vi "_GUI Template.vi"(8 "error in":errorcluster) -> (0 "error out":errorcluster)   [LabVIEW 2010]
doc: "GUI"
uses:
  <vilib>/Utility/miscctls.llb/LVPointTypeDef.ctl
panel:
  in  "Cancel":bool
  in  "OK":bool
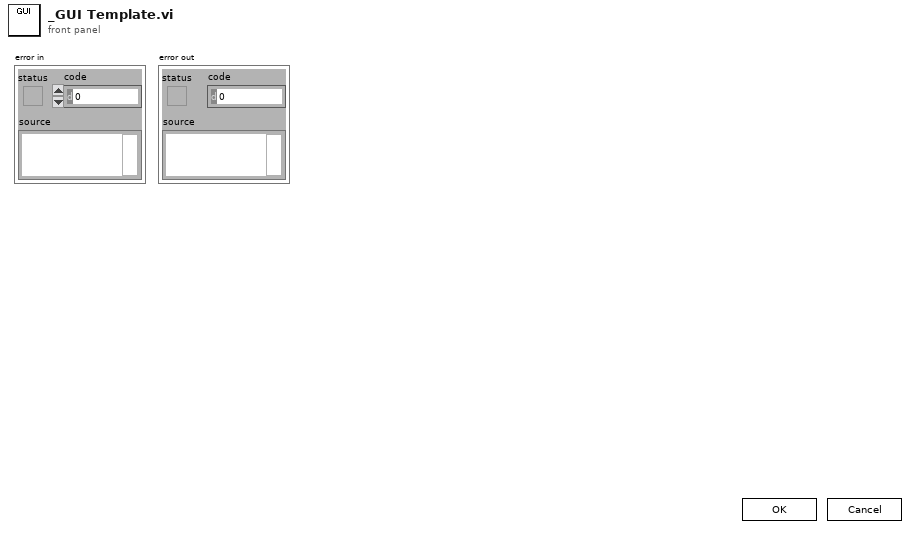
[diagram p1: front panel]
types:
  T1 = typedef "LVPointTypeDef.ctl" = cluster{"Horizontal":i16, "Vertical":i16}
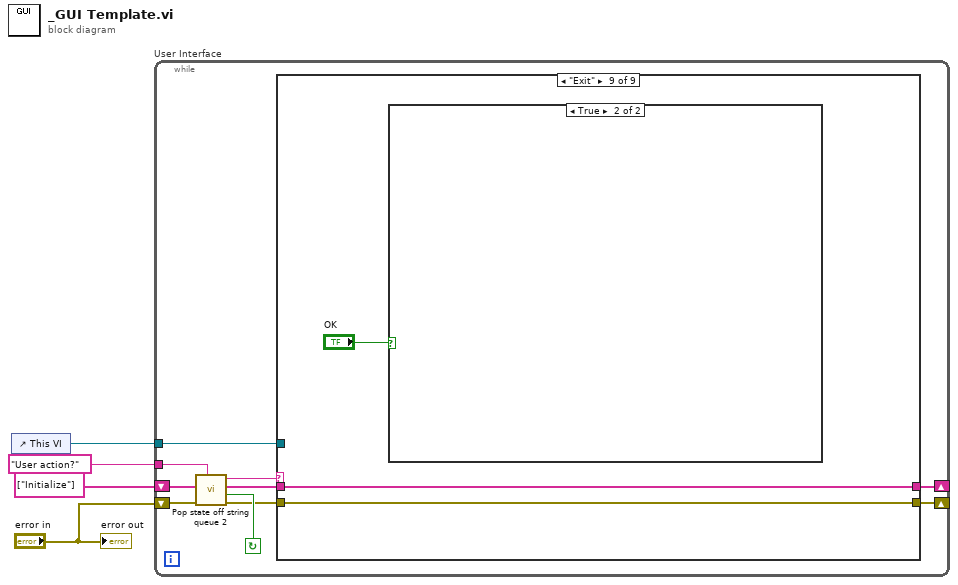
[diagram p0: block diagram]
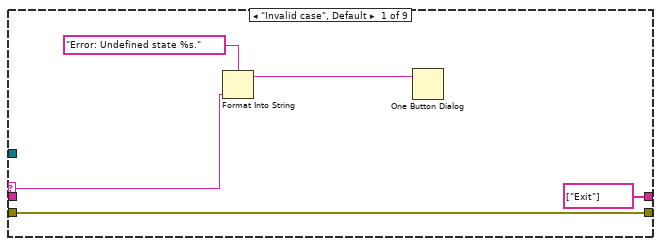
[diagram p2: hidden frame]
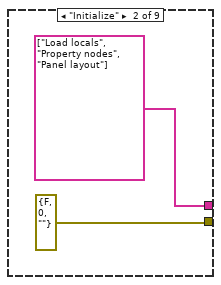
[diagram p3: hidden frame]
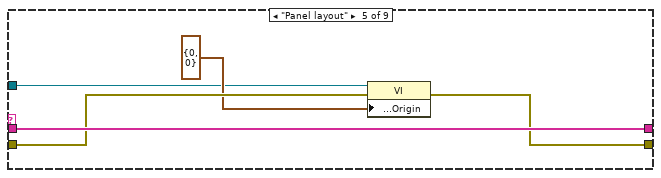
[diagram p6: hidden frame]
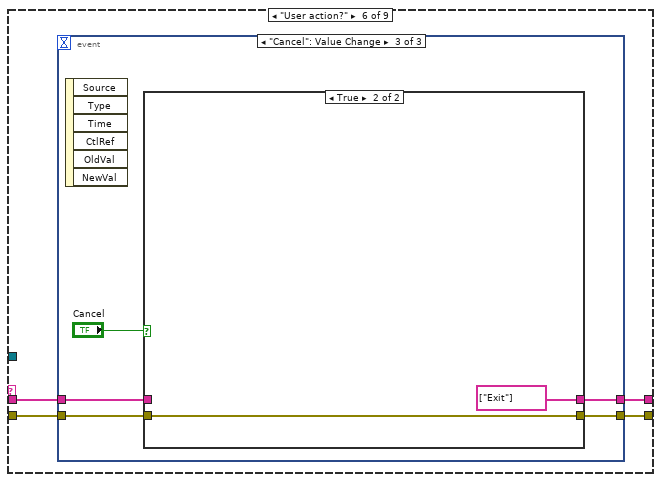
[diagram p7: hidden frame]
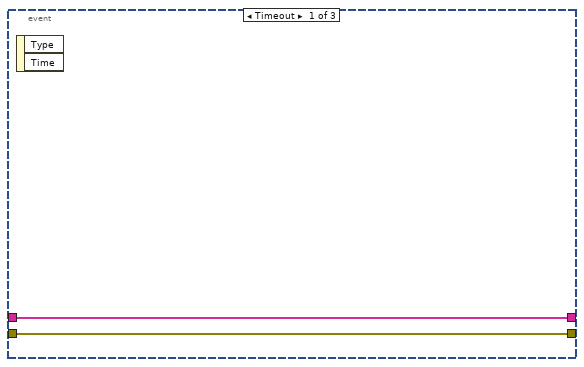
[diagram p8: hidden frame]
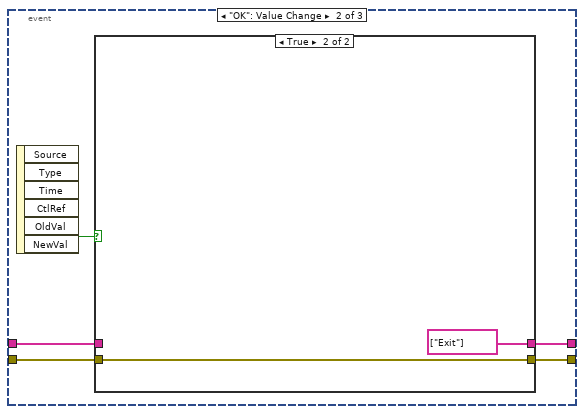
[diagram p9: hidden frame]
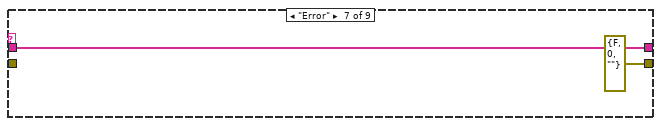
[diagram p12: hidden frame]
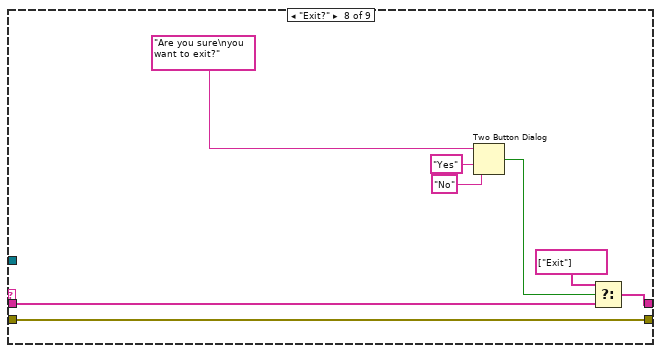
[diagram p13: hidden frame]
diagram:
  n1 = control-ref of="This VI"() -> (w2:refnum<vi>)
  n2 = while "User Interface" {
    shift-right: [w11] -> _
    shift-left: "error in" -> [w13]
    tunnel: "User action?" ("Default state") -> [w9]
    shift-right: [w8] -> _
    shift-left: string[] ["Initialize"] ("State que in") -> [w10]
    tunnel: w2 -> [w5]
    stop <- w14 continue-if-true
    n3 = call "Pop state off string queue 2.vi"("Default state"=w9, "error in (no error)"=w13, "State que in"=w10) -> ("error out"=w12:errorcluster, "Not Exit?"=w14:bool, "State que out"=w7:string[], "State case"=w6:string)  [unwired: 5 in]
    n4 = case shown="\"Exit\"" w6 {
      selector: w6 -> [w15 _ _ _ _ _ _ _ _]
      tunnel: w12 -> [w19 _ w23 w25 w28 w34 _ w64 w66]
      tunnel: [w19 errorcluster {"status"=FALSE, "code"=0, "source"=""} ("error out") w23 w25 w29 w33 errorcluster {"status"=FALSE, "code"=0, "source"=""} ("error out") w64 w66] -> w11
      tunnel: [string[] ["Exit"] ("State que in") string[] ["Load locals", "Property nodes", "Panel layout"] ("State que in") w22 w24 w30 w31 w56 w62 w67] -> w8
      tunnel: w7 -> [_ _ w22 w24 w30 w32 w56 w63 w67]
      tunnel: w5 -> [_ _ _ _ w26 _ _ _ _]
      frame "Invalid case", Default {
        n5 = Format Into String(format string="Error: Undefined state %s.", w15) -> (resulting string=w16:string)  [unwired: 2 in, 1 out]
        n6 = One Button Dialog(message=w16) -> ()  [unwired: 2 out]
      }
      frame "Initialize" {
      }
      frame "Load locals" {
      }
      frame "Property nodes" {
      }
      frame "Panel layout" {
        n7 = property class="VI"(reference=w26, error in=w28, "Front Panel Window:Origin"=T1 {"Horizontal"=0, "Vertical"=0}) -> (error out=w29:errorcluster)  [unwired: 1 out]
      }
      frame "User action?" {
        n8 = event shown="[2] \"Cancel\": Value Change" {
          selector: _ -> [_ _ _]
          dyn-events: _ -> [_ _ _]
          timeout: _ -> [_ _ _]
          tunnel: w34 -> [w36 w40 w49]
          tunnel: [w36 w39 w48] -> w33
          tunnel: w32 -> [w35 w41 w50]
          tunnel: [w35 w38 w47] -> w31
          event Timeout {
            n9 = event-data() -> ()  [unwired: 3 out]
          }
          event "OK": Value Change {
            n10 = event-data() -> ("NewVal"=w37:bool)  [unwired: 6 out]
            n11 = case shown="True" w37 {
              tunnel: w41 -> [w42 _]
              tunnel: w40 -> [w43 w45]
              tunnel: [w43 w45] -> w39
              tunnel: [w42 string[] ["Exit"] ("State que in")] -> w38
              frame False {
              }
              frame True {
              }
            }
          }
          event "Cancel": Value Change {
            n12 = event-data() -> ()  [unwired: 7 out]
            n13 = case shown="True" "Cancel" {
              tunnel: w50 -> [w51 _]
              tunnel: w49 -> [w52 w54]
              tunnel: [w52 w54] -> w48
              tunnel: [w51 string[] ["Exit"] ("State que in")] -> w47
              frame False {
              }
              frame True {
              }
            }
          }
        }
      }
      frame "Error" {
      }
      frame "Exit?" {
        n14 = Two Button Dialog(message="Are you sure\nyou want to exit?", 1:"No" ("F button name (\"Cancel\")"), 2:"Yes" ("T button name (\"OK\")")) -> (T button?=w58:bool)
        n15 = Select(t=string[] ["Exit"] ("State que out"), s=w58, f=w63) -> (s? t:f=w62:string[])
      }
      frame "Exit" {
        n16 = case shown="True" "OK" {
          frame False {
          }
          frame True {
          }
        }
      }
    }
  }
  "error out" <- "error in"
